vi "Monitor RefrigCapacity.vi"(8 "error in (no error)":errorcluster, 10 "Address (0)":i32, 11 "VISA resource name":refnum<visa-resource-name>) -> (0 "error out":errorcluster, 1 "Automatic":bool, 2 "Refrigerator SetPoint":u8, 3 "VISA resource name out":refnum<visa-resource-name>)   [LabVIEW 2016, in "Environment Chamber.lvlib" / "Climatic Chamber.lvlib"]
doc: "<b>Refrigerator setting monitor</b>\n\nReturns the refrigerator set point of the chamber.\n\n<b>P200:</B>\nSet point 0: Manual OFF (Stop)\nSet point 1: Manual ON\nSet point 2 to 9: Auto\n\n<b>SCP-220, P300:</B>\nSet point 0: Manual OFF (Stop)\nSet point 1 to 2: Manual 20% (Output: Small)\nSet point 3 to 5: Manual 50% (Output: Medium)\nSet point 6 to 8: Manual 100% (Max. Output)\nSet point 9: Auto"
uses:
  Climatic Chamber.lvlib
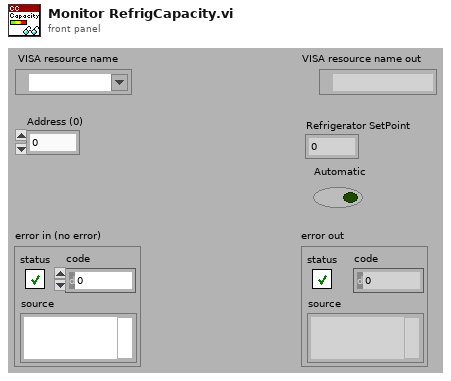
[diagram p1: front panel]
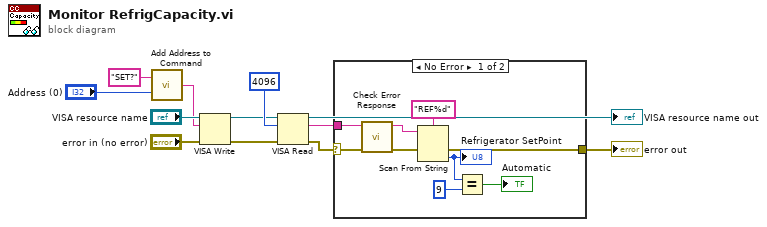
[diagram p0: block diagram]
diagram:
  n1 = call "Add Address to Command.vi"("Address (0)"="Address (0)", "Command"="SET?") -> ("Command OUT"=w5:string)
  n2 = VISA Write(VISA resource name="VISA resource name", write buffer=w5, error in (no error)="error in (no error)") -> (VISA resource name out=w9:refnum<visa-resource-name>, error out=w8:errorcluster)  [unwired: 1 out]
  n3 = VISA Read(VISA resource name=w9, byte count=u32 4096, error in (no error)=w8) -> (VISA resource name out=→"VISA resource name out":refnum<visa-resource-name>, read buffer=w3:string, error out=w4:errorcluster)  [unwired: 1 out]
  n4 = case shown="No Error" w4 {
    selector: w4 -> [w20 w22]
    tunnel: w3 -> [w21 _]
    tunnel: [w17 w22] -> w2
    frame No Error {
      n5 = call "Check Error Response.vi"("error in (no error)"=w20, "read String"=w21) -> ("error out"=w18:errorcluster, "String out"=w16:string)  [unwired: 7 in, 1 out]
      n6 = Scan From String(format string="REF%d", input string=w16, error in=w18) -> (error out=w17:errorcluster, output 1=w15:u8)  [unwired: 2 in, 2 out]
      "Refrigerator SetPoint" <- w15
      n7 = Equal?(x=w15, y=u8 9) -> (x = y?=→"Automatic":bool)
    }
    frame Error {
    }
  }
  "error out" <- w2
